vi "Table-TripleClick.vi"() -> ()   [LabVIEW 2013]
uses:
  <vilib>/event_ctls.llb/eventsource.ctl
  <vilib>/event_ctls.llb/lveventtype.ctl
  <vilib>/Utility/miscctls.llb/LVPoint32TypeDef.ctl
  <vilib>/Utility/miscctls.llb/LVRowAndColumnTypeDef.ctl
  <vilib>/Utility/cursorutil.llb/Set Cursor (Icon Pict).vi
panel:
  in  "String 2":string
  in  "String":string
  in  "Discard + string control Table":string[][](table)
  out "Mouse Down Event":T5={"Source"=0, "Type"=enum."Value Change", "Time"=0, "CtlRef"=refnum, "Coords"={"Horizontal"=0, "Vertical"=0}, "Button"=0, "Mods"={"Double Click"=FALSE, "Menu Key"=FALSE}, "PlatMods"={"Shift"=FALSE, "Ctrl"=FALSE, "Alt"=FALSE, "Cmd"=FALSE, "Opt"=FALSE}, "Invoke: Coords to row-col"={"In Bounds?"=FALSE, "Cell Position"={"Row"=0, "Column"=0}}} {"Source" items=["LabVIEW UI"=0, "ActiveX"=1, "User Event"=25]}
  in  "Mouse Down Table":string[][](table)
  out "Edit Position":T4
  out "Mouse Down? Event":T5={"Source"=0, "Type"=enum."Value Change", "Time"=0, "CtlRef"=refnum, "Coords"={"Horizontal"=0, "Vertical"=0}, "Button"=0, "Mods"={"Double Click"=FALSE, "Menu Key"=FALSE}, "PlatMods"={"Shift"=FALSE, "Ctrl"=FALSE, "Alt"=FALSE, "Cmd"=FALSE, "Opt"=FALSE}, "Invoke: Coords to row-col"={"In Bounds?"=FALSE, "Cell Position"={"Row"=0, "Column"=0}}} {"Source" items=["LabVIEW UI"=0, "ActiveX"=1, "User Event"=25]}
  in  "Mouse Down? Table":string[][](table)
  in  "stop":bool
  in  "Simple Table":string[][](table)
  # "This table moves a string control depending on user clicks,\ndemonstrating how edit box could be self-handled...\nTriple click works, but lots of code needed to give same\nfunctionality table provides for free!"
  # "<--Triple click works.\nThere are NO click events handled for this simple table."
  # "<--Triple click does NOT works.\nWith a Mouse Down? event that simply chooses not to discard\nthe click, triple click is broken."
  # "When not using the filtering event, triple click still works!"
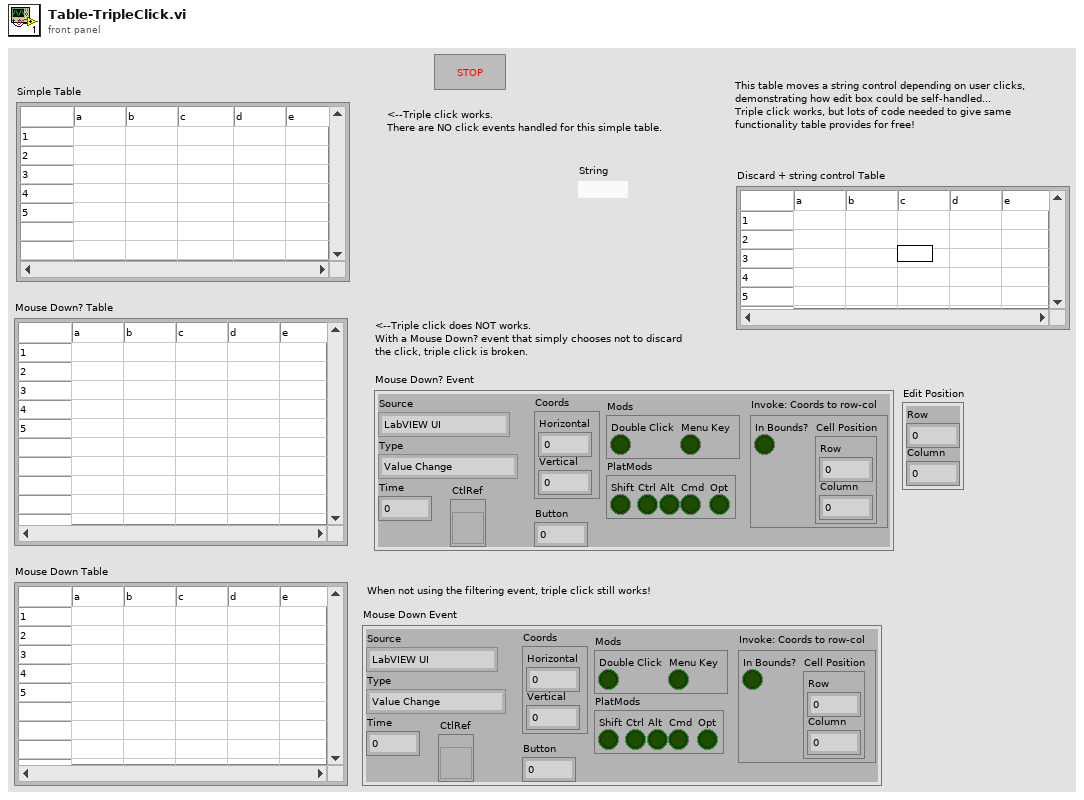
[diagram p1: front panel]
types:
  T1 = typedef "eventsource.ctl" = u32
  T2 = typedef "lveventtype.ctl" = enum32{"Null", "Timeout", "Annotation Menu Selection", "Annotation Menu Selection?", "App Instance Close", "App Instance Close?", "Autoscale Range Change", "Bookmark Info Change", "Cell Edit", "Cell Edit?", "Cursor Grab", "Cursor Grab?", "Cursor Menu Selection", "Cursor Menu Selection?", "Cursor Move", "Cursor Release", "Data Change", "Direction Change", "Display State Change", "Drag Ended", "Drag Enter", "Drag Leave", "Drag Over", "Drag Source Update", "Drag Starting", "Drag Starting?", "Drop", "Exec State Change", "Key Down", "Key Down?", "Key Repeat", "Key Repeat?", "Key Up", "Listbox Double Click", "Menu Activation?", "Menu Selection (App)", "Menu Selection? (App)", "Menu Selection (User)", "Mouse Down", "Mouse Down?", "Mouse Enter", "Mouse Leave", "Mouse Move", "Mouse Up", "Mouse Wheel", "NI Security User Change (App)", "Pane Size", "Panel Close", "Panel Close?", "Panel Resize", "Plot Attribute Change", "Scale Range Change", "Shortcut Menu Activation?", "Shortcut Menu Selection (App)", "Shortcut Menu Selection? (App)", "Shortcut Menu Selection (User)", "Tree Double Click", "Tree Drag", "Tree Drag?", "Tree Drop", "Tree Drop?", "Tree Item Close", "Tree Item Close?", "Tree Item Open", "Tree Item Open?", "User Event", "Value Change"}
  T3 = typedef "LVPoint32TypeDef.ctl" = cluster{"Horizontal":i32, "Vertical":i32}
  T4 = typedef "LVRowAndColumnTypeDef.ctl" = cluster{"Row":i32, "Column":i32}
  T5 = cluster{"Source":T1, "Type":T2, "Time":u32, "CtlRef":refnum<vi>, "Coords":T3, "Button":u16, "Mods":cluster{"Double Click":bool, "Menu Key":bool}, "PlatMods":cluster{"Shift":bool, "Ctrl":bool, "Alt":bool, "Cmd":bool, "Opt":bool}, "Invoke: Coords to row-col":cluster{"In Bounds?":bool, "Cell Position":T4}}
  T6 = cluster{"Shift":bool, "Ctrl":bool, "Alt":bool, "Cmd":bool, "Opt":bool}
  T7 = typedef "LVPositionTypeDef.ctl" = cluster{"Left":i32, "Top":i32}
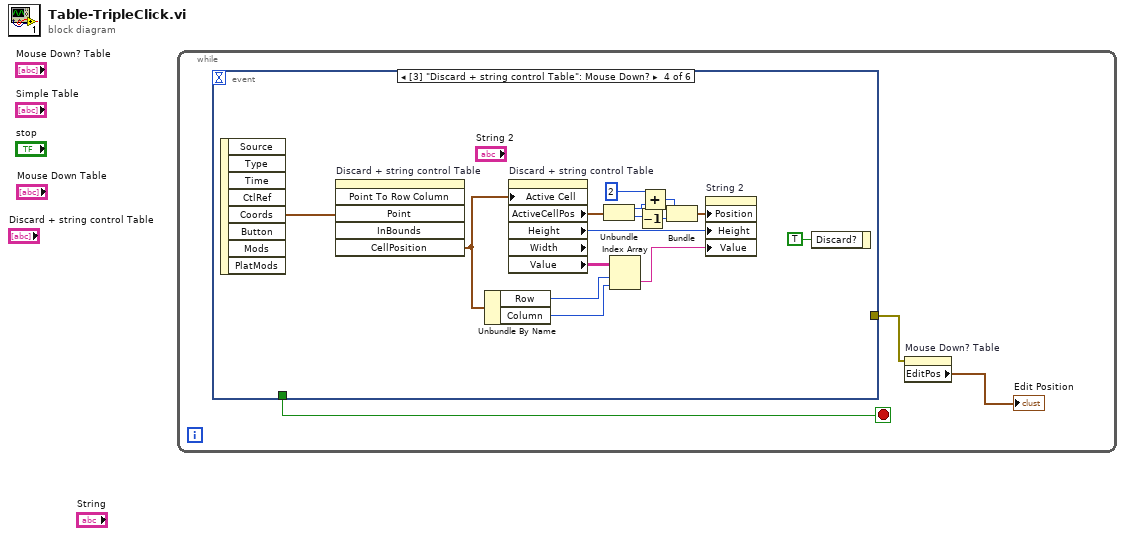
[diagram p0: block diagram]
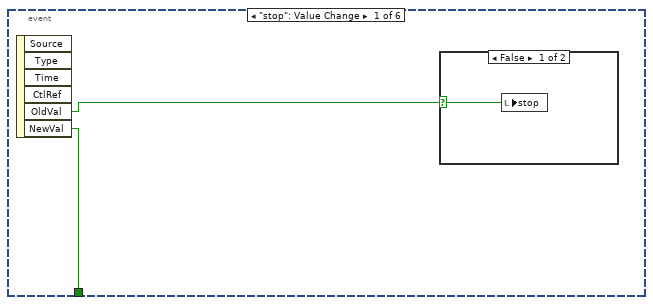
[diagram p2: hidden frame]
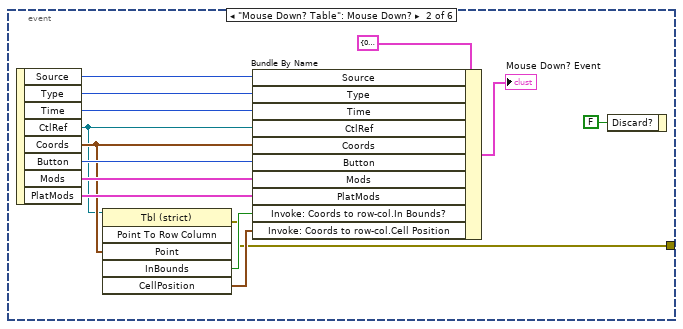
[diagram p4: hidden frame]
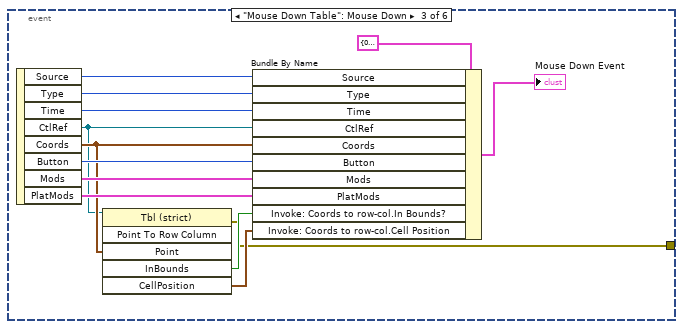
[diagram p5: hidden frame]
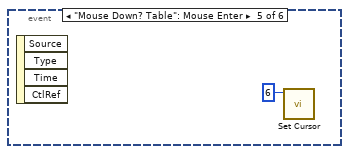
[diagram p6: hidden frame]
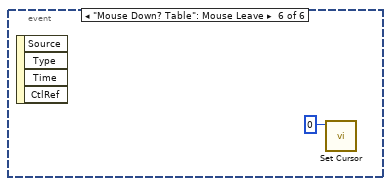
[diagram p7: hidden frame]
diagram:
  n1 = while {
    stop <- w3 stop-if-true
    n2 = event shown="[3] \"Discard + string control Table\": Mouse Down?" {
      selector: _ -> [_ _ _ _ _ _]
      dyn-events: _ -> [_ _ _ _ _ _]
      timeout: _ -> [_ _ _ _ _ _]
      tunnel: [w5 _ _ _ _ _] -> w3
      tunnel: [_ w7 w22 _ _ _] -> w1
      event "stop": Value Change {
        n3 = event-data() -> ("OldVal"=w4:bool, "NewVal"=w5:bool)  [unwired: 1 in, 4 out]
        n4 = case shown="False" w4 {
          selector: w4 -> [w6 _]
          frame False {
            n5 = local write "stop"(w6) -> ()
          }
          frame True {
          }
        }
      }
      event "Mouse Down? Table": Mouse Down? {
        n6 = event-data() -> ("Source"=w18:T1, "Type"=w17:T2, "Time"=w16:u32, "CtlRef"=w9:refnum<vi>, "Coords"=w11:T3, "Button"=w15:u16, "Mods"=w14:cluster{"Double Click":bool, "Menu Key":bool}, "PlatMods"=w13:T6)  [unwired: 1 in]
        n7 = invoke class="Tbl (strict)" method="Point To Row Column"(reference=w9, "Point"=w11) -> (error out=w7:errorcluster, "InBounds"=w10:bool, "CellPosition"=w8:T4)  [unwired: 4 in, 3 out]
        n8 = Bundle By Name(cluster=T5 {"Source"=0, "Type"=enum."Value Change", "Time"=0, "CtlRef"=refnum, "Coords"={"Horizontal"=0, "Vertical"=0}, "Button"=0, "Mods"={"Double Click"=FALSE, "Menu Key"=FALSE}, "PlatMods"={"Shift"=FALSE, "Ctrl"=FALSE, "Alt"=FALSE, "Cmd"=FALSE, "Opt"=FALSE}, "Invoke: Coords to row-col"={"In Bounds?"=FALSE, "Cell Position"={"Row"=0, "Column"=0}}} ("Mouse Down Event"), "Source"=w18, "Type"=w17, "Time"=w16, "CtlRef"=w9, "Coords"=w11, "Button"=w15, "Mods"=w14, "PlatMods"=w13, "Invoke: Coords to row-col.In Bounds?"=w10, "Invoke: Coords to row-col.Cell Position"=w8) -> (→"Mouse Down? Event":T5)
        n9 = event-data("Discard?"=FALSE) -> ()  [unwired: 1 in, 1 out]
      }
      event "Mouse Down Table": Mouse Down {
        n10 = event-data() -> ("Source"=w32:T1, "Type"=w31:T2, "Time"=w30:u32, "CtlRef"=w24:refnum<vi>, "Coords"=w26:T3, "Button"=w29:u16, "Mods"=w28:cluster{"Double Click":bool, "Menu Key":bool}, "PlatMods"=w27:T6)  [unwired: 1 in]
        n11 = invoke class="Tbl (strict)" method="Point To Row Column"(reference=w24, "Point"=w26) -> (error out=w22:errorcluster, "InBounds"=w25:bool, "CellPosition"=w23:T4)  [unwired: 4 in, 3 out]
        n12 = Bundle By Name(cluster=T5 {"Source"=0, "Type"=enum."Value Change", "Time"=0, "CtlRef"=refnum, "Coords"={"Horizontal"=0, "Vertical"=0}, "Button"=0, "Mods"={"Double Click"=FALSE, "Menu Key"=FALSE}, "PlatMods"={"Shift"=FALSE, "Ctrl"=FALSE, "Alt"=FALSE, "Cmd"=FALSE, "Opt"=FALSE}, "Invoke: Coords to row-col"={"In Bounds?"=FALSE, "Cell Position"={"Row"=0, "Column"=0}}} ("Mouse Down Event"), "Source"=w32, "Type"=w31, "Time"=w30, "CtlRef"=w24, "Coords"=w26, "Button"=w29, "Mods"=w28, "PlatMods"=w27, "Invoke: Coords to row-col.In Bounds?"=w25, "Invoke: Coords to row-col.Cell Position"=w23) -> (→"Mouse Down Event":T5)
      }
      event "Discard + string control Table": Mouse Down? {
        n13 = event-data() -> ("Coords"=w47:T3)  [unwired: 1 in, 7 out]
        n14 = invoke on="Discard + string control Table" class="Tbl (strict)" method="Point To Row Column"("Point"=w47) -> ("CellPosition"=w45:T4)  [unwired: 5 in, 5 out]
        n15 = Unbundle By Name(w45) -> ("Row"=w43:i32, "Column"=w42:i32)
        n16 = property on="Discard + string control Table" class="Tbl (strict)" props=["Active Cell", "ActiveCellPos", "Height", "Width", "Value"]("Active Cell"=w45) -> ("ActiveCellPos"=w40:T7, "Height"=w46:u32, "Value"=w44:string[][])  [unwired: 2 in, 3 out]
        n17 = Unbundle(w40) -> ("Left"=w38:i32, "Top"=w35:i32)
        n18 = Index Array(array=w44, index (row)=w43, index (col)=w42) -> (element=w41:string)
        n19 = Decrement(x=w35) -> (x-1=w34:i32)
        n20 = Add(x=2, y=w38) -> (x+y=w37:i32)
        n21 = Bundle(w37, w34) -> (w39:cluster{i32, i32})  [unwired: 1 in]
        n22 = property on="String 2" class="Str"("Position"=w39, "Height"=w46, "Value"=w41) -> ()  [unwired: 2 in, 2 out]
        n23 = event-data("Discard?"=TRUE) -> ()  [unwired: 1 in, 1 out]
      }
      event "Mouse Down? Table": Mouse Enter {
        n24 = event-data() -> ()  [unwired: 1 in, 4 out]
        n25 = call-poly <vilib>:"Set Cursor.vi"("icon"=u16 6) -> ()  [unwired: 9 in, 2 out]
      }
      event "Mouse Down? Table": Mouse Leave {
        n26 = event-data() -> ()  [unwired: 1 in, 4 out]
        n27 = call-poly <vilib>:"Set Cursor.vi"("icon"=u16 0) -> ()  [unwired: 9 in, 2 out]
      }
    }
    n28 = property on="Mouse Down? Table" class="Tbl (strict)"(error in=w1) -> ("EditPos"=→"Edit Position":T4)  [unwired: 1 in, 2 out]
  }
